vi "CMD_RSM - SE4500 - Poke PRISM Register GENERIC command.vi"(0 "Input_Data":string[](array[string]), 5 "Error In":errorcluster) -> (12 "Validate CheckSum":bool, 13 "Command":u8[](array[numeric])=[4, 228, 4, 128, 0, 0, 0, 0, 0, 0, 0, 0, 0, 0] format="%x", 14 "Response":bool, 15 "Ack":bool, 16 "Command":bool, 17 "Add CheckSum":bool, 18 "Status":bool, 19 "Error Out":errorcluster)   [LabVIEW 2014]
panel:
  # "Flags"
  # "RSM - SE4500 - Poke PRISM Register GENERIC command:"
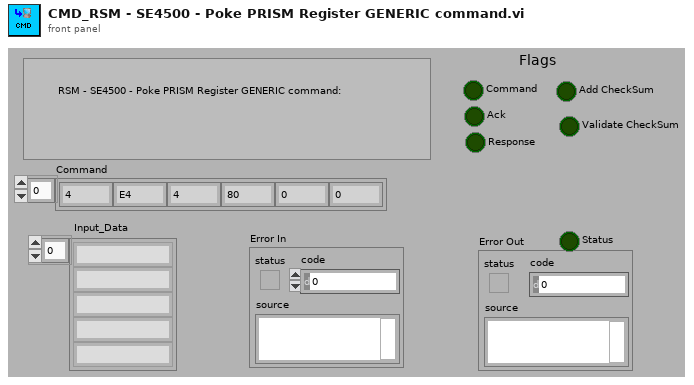
[diagram p1: front panel]
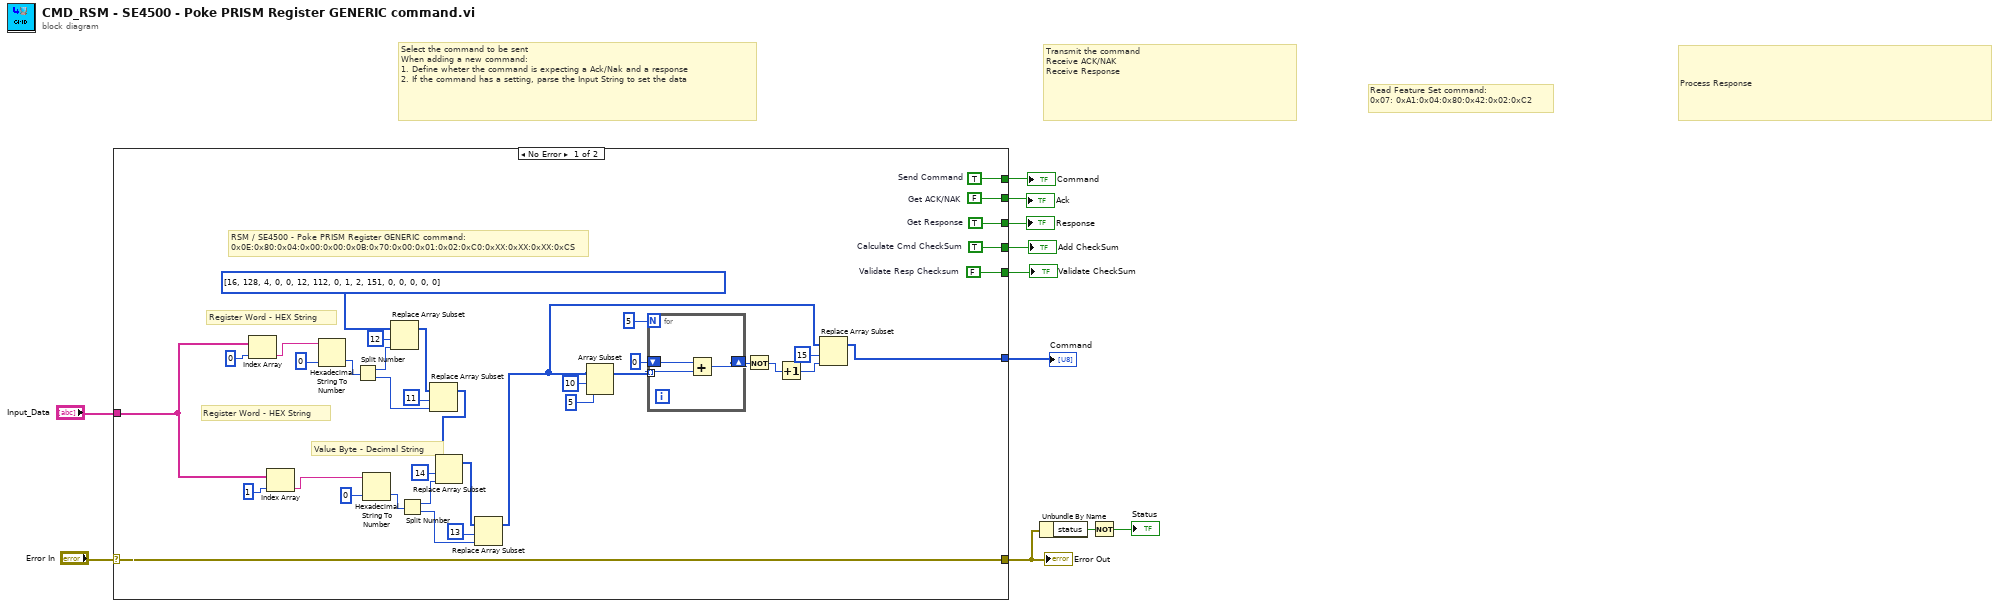
[diagram p0: block diagram]
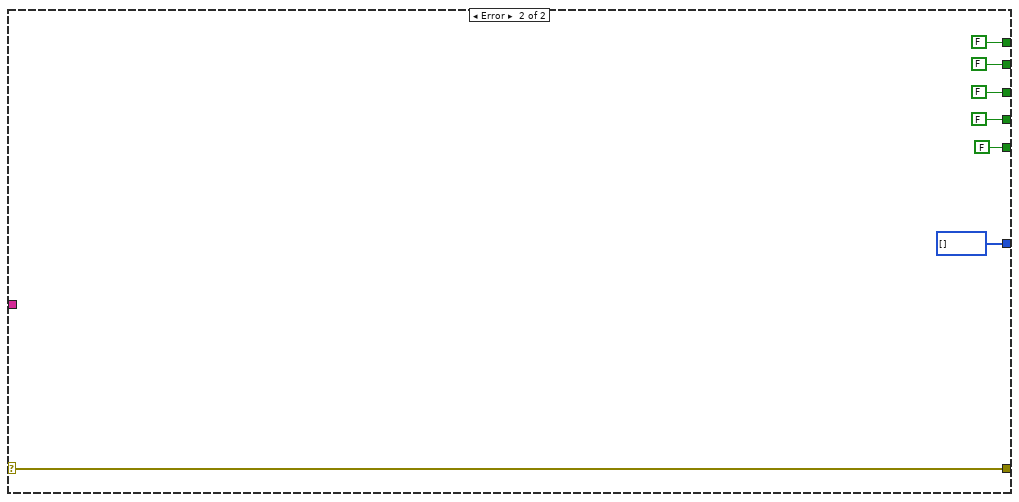
[diagram p2: hidden frame]
diagram:
  # "Read Feature Set command:\n0x07: 0xA1:0x04:0x80:0x42:0x02:0xC2"
  # "Process Response"
  # "Transmit the command\nReceive ACK/NAK\nReceive Response"
  # "Select the command to be sent\nWhen adding a new command:\n1. Define wheter the command is expecting a Ack/Nak and a response\n2. If the command has a setting, parse the Input String to set the data"
  n1 = case shown="No Error" "Error In" {
    selector: "Error In" -> [w45 w54]
    tunnel: [w49 FALSE ("Send Command")] -> w10
    tunnel: [w48 FALSE ("Get ACK/NAK")] -> w9
    tunnel: [w47 FALSE ("Get Response")] -> w8
    tunnel: [w46 FALSE ("Add CheckSum")] -> w7
    tunnel: [w12 u8[] []] -> w6
    tunnel: [w45 w54] -> w4
    tunnel: "Input_Data" -> [w13 _]
    tunnel: [w44 FALSE ("Validate Resp Checksum")] -> w1
    frame No Error {
      w44 = FALSE  # Validate Resp Checksum
      w46 = TRUE  # Calculate Cmd CheckSum
      w47 = TRUE  # Get Response
      w49 = TRUE  # Send Command
      w48 = FALSE  # Get ACK/NAK
      # "Register Word - HEX String"
      # "Register Word - HEX String"
      # "Value Byte - Decimal String"
      # "RSM / SE4500 - Poke PRISM Register GENERIC command:\n0x0E:0x80:0x04:0x00:0x00:0x0B:0x70:0x00:0x01:0x02:0xC0:0xXX:0xXX:0xXX:0xCS"
      n2 = Index Array(array=w13, index=0) -> (element=w27:string)
      n3 = Index Array(array=w13, index=1) -> (element=w18:string)
      n4 = Hexadecimal String To Number(string=w27, default (0uL)=i16 0 ("default (0 I32)")) -> (number=w25:i16)  [unwired: 1 in, 1 out]
      n5 = Split Number(x=w25) -> (hi(x)=w31:u8, lo(x)=w29:u8)
      n6 = Hexadecimal String To Number(string=w18, default (0uL)=i16 0 ("default (0 I32)")) -> (number=w24:i16)  [unwired: 1 in, 1 out]
      n7 = Replace Array Subset(array=u8[] [16, 128, 4, 0, 0, 12, 112, 0, 1, 2, 151, 0, 0, 0, 0, 0], new element=w31, index=12) -> (w28:u8[])
      n8 = Split Number(x=w24) -> (hi(x)=w21:u8, lo(x)=w23:u8)
      n9 = Replace Array Subset(array=w28, new element=w29, index=11) -> (w16:u8[])
      n10 = Replace Array Subset(array=w16, new element=w21, index=14) -> (w15:u8[])
      n11 = Replace Array Subset(array=w15, new element=w23, index=13) -> (w14:u8[])
      n12 = Array Subset(array=w14, index=10, length=5) -> (w34:u8[])
      n13 = for {
        N: 5 -> [_]
        tunnel: w34 -> [w52] mode=indexing
        shift-right: [w50] -> w40
        shift-left: u16 0 -> [w51]
        n14 = Add(x=w51, y=w52) -> (x+y=w50:u16)
      }
      n15 = Not(x=w40) -> (.not. x?=w39:u16)
      n16 = Increment(x=w39) -> (x+1=w38:u16)
      n17 = Replace Array Subset(array=w14, new element=w38, index=15) -> (w12:u8[])
    }
    frame Error {
    }
  }
  "Error Out" <- w4
  "Command" <- w10
  "Ack" <- w9
  "Response" <- w8
  "Add CheckSum" <- w7
  "Command" <- w6
  "Validate CheckSum" <- w1
  n18 = Unbundle By Name(w4) -> ("status"=w3:bool)
  n19 = Not(x=w3) -> (.not. x?=→"Status":bool)
